vi "Test Summary Page.vi"(8 "error in (no error)":errorcluster, 9 "Test Configuration":T1, 10 "Test Results":T8, 11 "Type":string="Step") -> (0 "error out":errorcluster, 3 "Result":bool)   [LabVIEW 2015]
uses:
  Tests/Controls/Test Results.ctl
  Tests/Controls/Step Result.ctl
  Tests/Controls/Test Configuration.ctl
  Tests/Controls/Vacuum Test.ctl
  Tests/Controls/Test Timing.ctl
  Tests/Controls/Vaccum Thresholds.ctl
  Tests/Controls/Helium Test.ctl
  Tests/Controls/Helium Thresholds.ctl
  Tests/Controls/Functional Test.ctl
panel:
  out "String Result":string
  in  "OK":bool
  in  "Thresholds":i32(listbox)=-1
  # "Test Result Summary"
  # "Result"
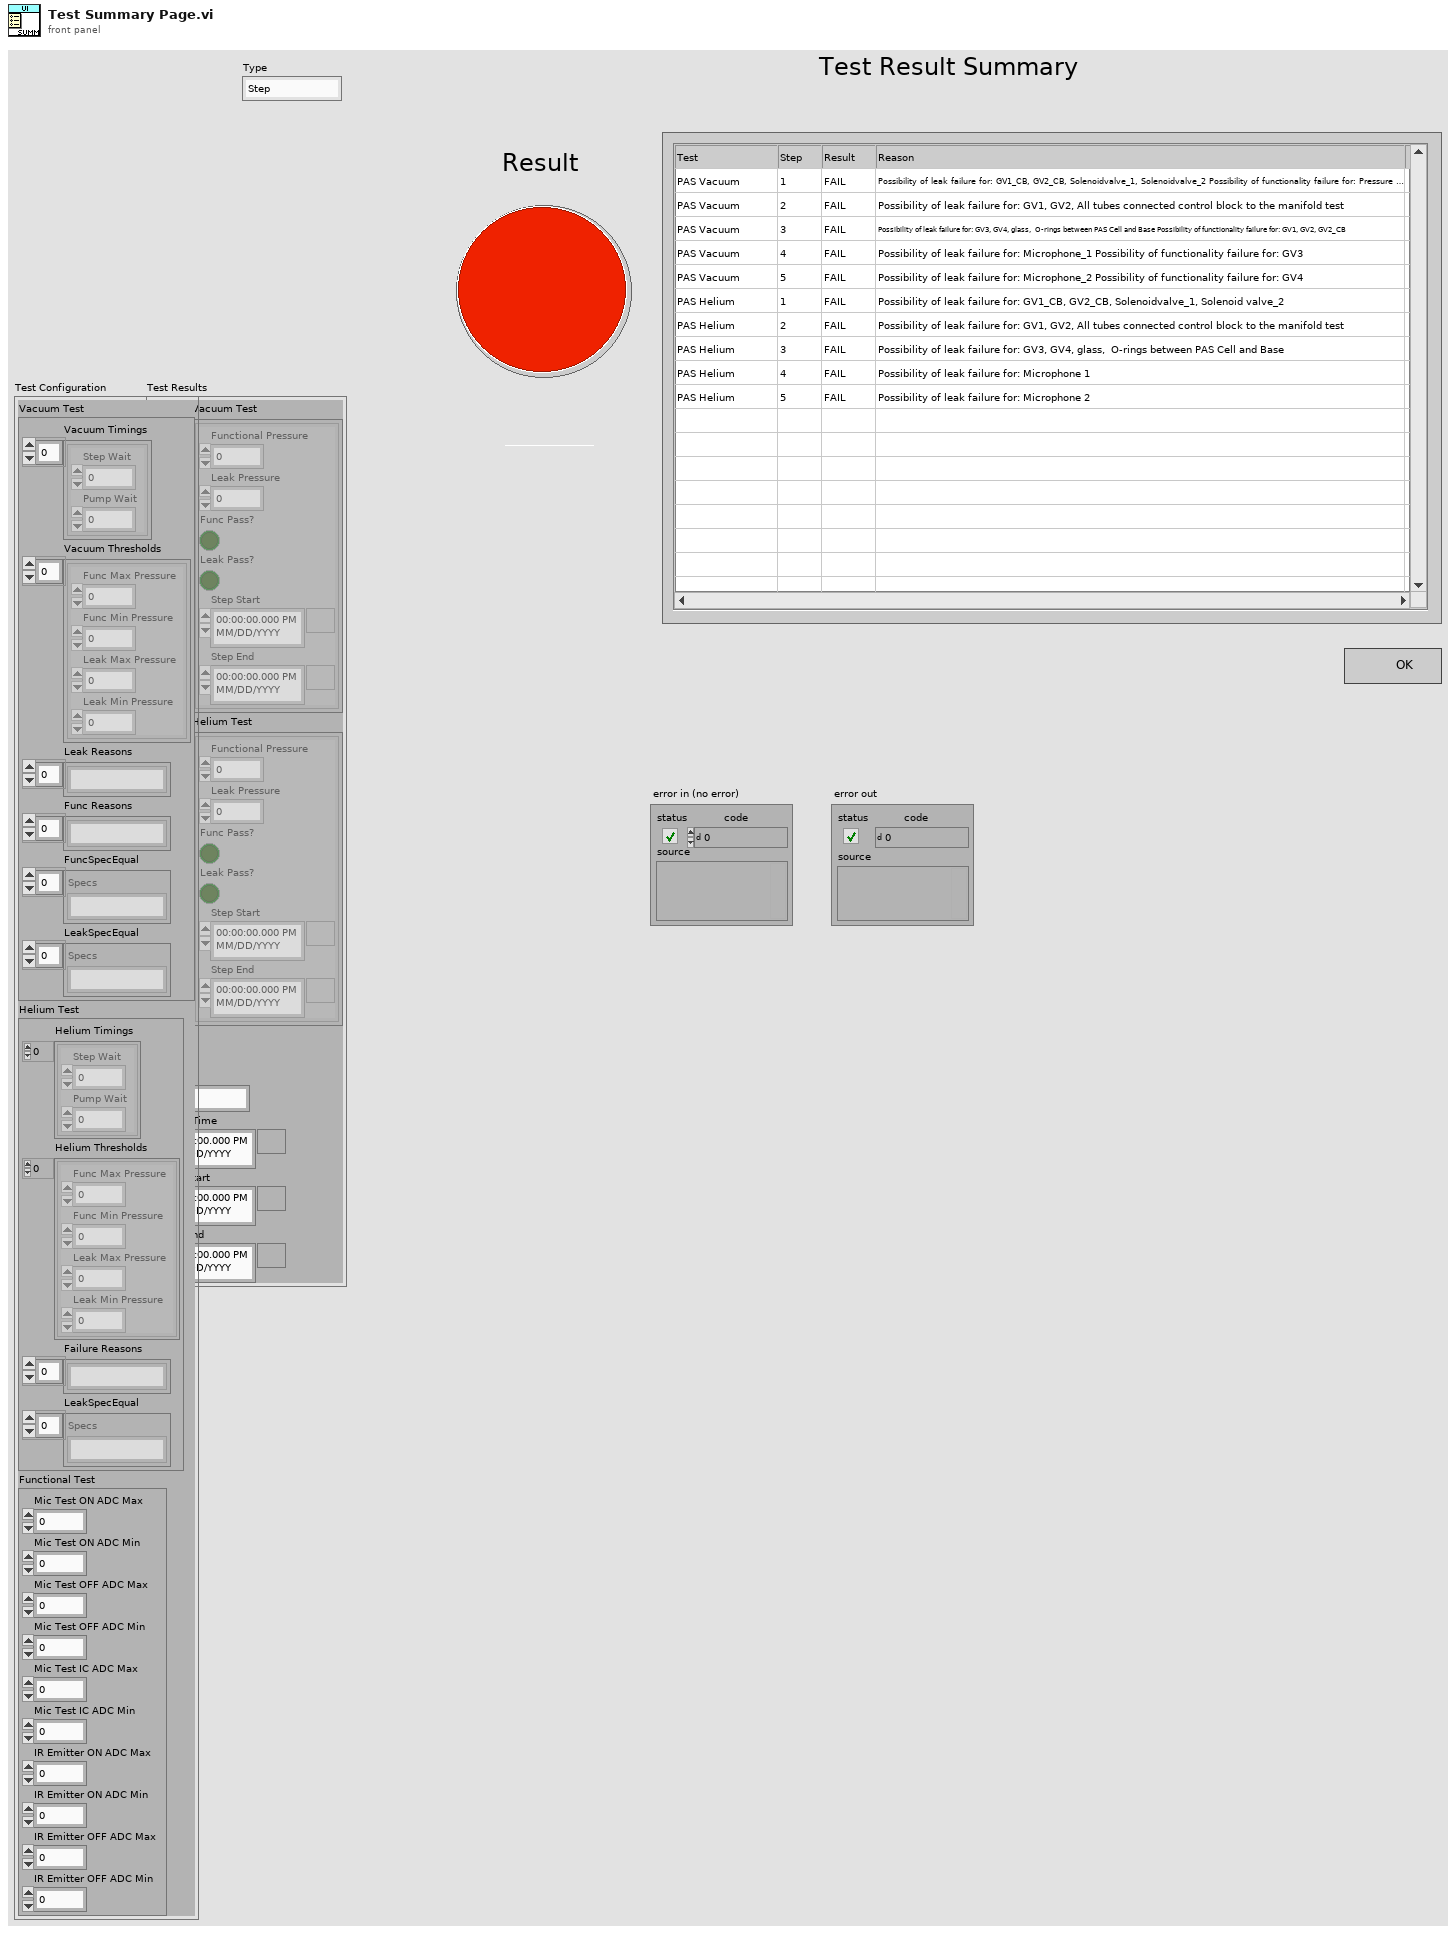
[diagram p1: front panel]
types:
  T1 = typedef "Test Configuration.ctl" = cluster{"Vacuum Test":T2, "Helium Test":T5, "Functional Test":T7}
  T2 = typedef "Vacuum Test.ctl" = cluster{"Vacuum Timings":T3[], "Vacuum Thresholds":T4[], "Leak Reasons":string[], "Func Reasons":string[], "FuncSpecEqual":string[], "LeakSpecEqual":string[]}
  T3 = typedef "Test Timing.ctl" = cluster{"Step Wait":dbl, "Pump Wait":dbl}
  T4 = typedef "Vaccum Thresholds.ctl" = cluster{"Func Max Pressure":dbl, "Func Min Pressure":dbl, "Leak Max Pressure":dbl, "Leak Min Pressure":dbl}
  T5 = typedef "Helium Test.ctl" = cluster{"Helium Timings":T3[], "Helium Thresholds":T6[], "Failure Reasons":string[], "LeakSpecEqual":string[]}
  T6 = typedef "Helium Thresholds.ctl" = cluster{"Func Max Pressure":dbl, "Func Min Pressure":dbl, "Leak Max Pressure":dbl, "Leak Min Pressure":dbl}
  T7 = typedef "Functional Test.ctl" = cluster{"Mic Test ON ADC Max":dbl, "Mic Test ON ADC Min":dbl, "Mic Test OFF ADC Max":dbl, "Mic Test OFF ADC Min":dbl, "Mic Test IC ADC Max":dbl, "Mic Test IC ADC Min":dbl, "IR Emitter ON ADC Max":dbl, "IR Emitter ON ADC Min":dbl, "IR Emitter OFF ADC Max":dbl, "IR Emitter OFF ADC Min":dbl}
  T8 = typedef "Test Results.ctl" = cluster{"Vacuum Test":T9[], "Helium Test":T9[], "Aborted?":bool, "Reason":string, "Abort Time":timestamp, "Test Start":timestamp, "Test End":timestamp}
  T9 = typedef "Step Result.ctl" = cluster{"Functional Pressure":dbl, "Leak Pressure":dbl, "Func Pass?":bool, "Leak Pass?":bool, "Step Start":timestamp, "Step End":timestamp}
  T10 = typedef "LVPoint32TypeDef.ctl" = cluster{"Horizontal":i32, "Vertical":i32}
  T11 = typedef "LVRowAndColumnTypeDef.ctl" = cluster{"Row":i32, "Column":i32}
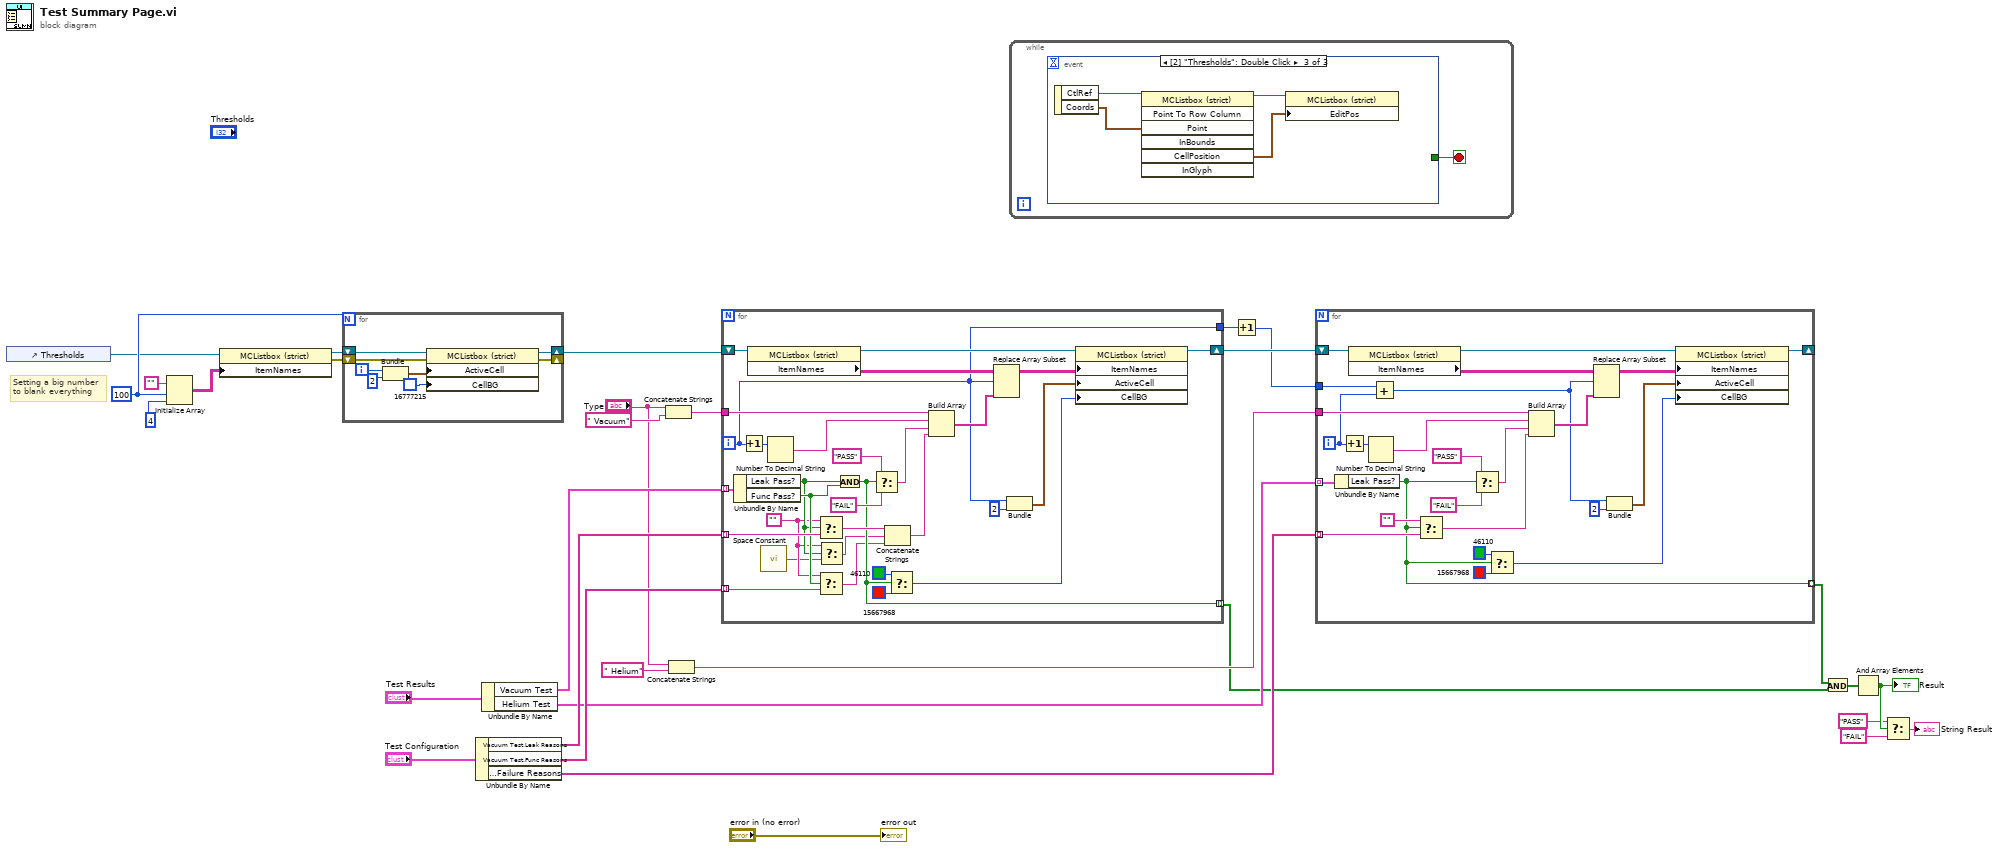
[diagram p0: block diagram]
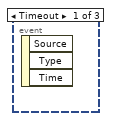
[diagram p2: hidden frame]
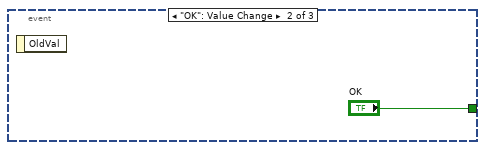
[diagram p3: hidden frame]
diagram:
  w8 = 100 ("dimension size")
  # "Setting a big number\nto blank everything"
  n1 = control-ref of="Thresholds"() -> (w7:refnum<vi>)
  n2 = Initialize Array("", w8, 4 ("dimension size")) -> (w12:string[][])
  n3 = property class="MCListbox (strict)"(reference=w7, "ItemNames"=w12) -> (reference out=w11:refnum<vi>, error out=w10:errorcluster)  [unwired: 1 in]
  n4 = for {
    N: w8 -> [_]
    shift-right: [w38] -> w6
    shift-left: w11 -> [w39]
    shift-right: [w32] -> _
    shift-left: w10 -> [w33]
    i -> [w37]
    n5 = Bundle(w37, "element"=2) -> (w35:cluster{i32, "element":i32})  [unwired: 1 in]
    n6 = property class="MCListbox (strict)"(reference=w39, error in=w33, "ActiveCell"=w35, "CellBG"=u32 16777215) -> (reference out=w38:refnum<vi>, error out=w32:errorcluster)
  }
  n7 = Unbundle By Name("Test Configuration") -> ("Vacuum Test.Leak Reasons"=w27:string[], "Vacuum Test.Func Reasons"=w26:string[], "Helium Test.Failure Reasons"=w21:string[])
  n8 = Unbundle By Name("Test Results") -> ("Vacuum Test"=w31:T9[], "Helium Test"=w22:T9[])
  n9 = Concatenate Strings("Type", " Vacuum") -> (w29:string)
  n10 = Concatenate Strings("Type", " Helium") -> (w23:string)
  n11 = for {
    tunnel: w31 -> [w69] mode=indexing
    tunnel: w29 -> [w65]
    tunnel: w27 -> [w62] mode=indexing
    tunnel: w26 -> [w60] mode=indexing
    shift-right: [w52] -> w25
    shift-left: w6 -> [w57]
    tunnel: [w46] -> w5 mode=indexing
    tunnel: [w45] -> w20
    i -> [w45]
    w42 = ""
    n12 = Unbundle By Name(w69) -> ("Leak Pass?"=w43:bool, "Func Pass?"=w61:bool)
    n13 = Increment(x=w45) -> (x+1=w68:i32)
    n14 = property class="MCListbox (strict)"(reference=w57) -> (reference out=w54:refnum<vi>, "ItemNames"=w56:string[][])  [unwired: 1 in, 1 out]
    n15 = call <vilib>:"Space Constant.vi"() -> ("String"=w41:string)
    n16 = Number To Decimal String(number=w68) -> (decimal integer string=w64:string)  [unwired: 1 in]
    n17 = Select(t=w42, s=w43, f=w62) -> (s? t:f=w59:string)
    n18 = Select(t=w42, s=w61, f=w60) -> (s? t:f=w44:string)
    n19 = Select(t=w42, s=w43, f=w41) -> (s? t:f=w40:string)
    n20 = And(x=w43, y=w61) -> (x .and. y?=w46:bool)
    n21 = Select(t="PASS", s=w46, f="FAIL") -> (s? t:f=w63:string)
    n22 = Concatenate Strings(w59, w40, w44) -> (w58:string)
    n23 = Select(t=u32 46110, s=w46, f=u32 15667968) -> (s? t:f=w47:u32)
    n24 = Build Array(w65, w64, w63, w58) -> (w55:string[])
    n25 = Replace Array Subset(array=w56, new element=w55, index (row)=w45) -> (w53:string[][])  [unwired: 1 in]
    n26 = Bundle(w45, 2) -> (w50:cluster{i32, i32})  [unwired: 1 in]
    n27 = property class="MCListbox (strict)"(reference=w54, "ItemNames"=w53, "ActiveCell"=w50, "CellBG"=w47) -> (reference out=w52:refnum<vi>)  [unwired: 1 in, 1 out]
  }
  n28 = while {
    stop <- w70 stop-if-true
    n29 = event shown="[2] \"Thresholds\": Double Click" {
      selector: _ -> [_ _ _]
      dyn-events: _ -> [_ _ _]
      timeout: _ -> [_ _ _]
      tunnel: [_ "OK" _] -> w70
      event Timeout {
        n30 = event-data() -> ()  [unwired: 1 in, 3 out]
      }
      event "OK": Value Change {
        n31 = event-data() -> ()  [unwired: 1 in, 1 out]
      }
      event "Thresholds": Double Click {
        n32 = event-data() -> ("CtlRef"=w75:refnum<vi>, "Coords"=w74:T10)  [unwired: 1 in]
        n33 = invoke class="MCListbox (strict)" method="Point To Row Column"(reference=w75, "Point"=w74) -> (reference out=w73:refnum<vi>, "CellPosition"=w72:T11)  [unwired: 5 in, 5 out]
        n34 = property class="MCListbox (strict)"(reference=w73, "EditPos"=w72) -> ()  [unwired: 1 in, 2 out]
      }
    }
  }
  n35 = Increment(x=w20) -> (x+1=w19:i32)
  n36 = for {
    tunnel: w22 -> [w100] mode=indexing
    tunnel: w23 -> [w96]
    tunnel: w21 -> [w93] mode=indexing
    shift-right: [w87] -> _
    shift-left: w25 -> [w92]
    tunnel: [w80] -> w18 mode=indexing
    tunnel: w19 -> [w78]
    i -> [w77]
    n37 = Unbundle By Name(w100) -> ("Leak Pass?"=w80:bool)
    n38 = Increment(x=w77) -> (x+1=w99:i32)
    n39 = property class="MCListbox (strict)"(reference=w92) -> (reference out=w89:refnum<vi>, "ItemNames"=w91:string[][])  [unwired: 1 in, 1 out]
    n40 = Number To Decimal String(number=w99) -> (decimal integer string=w95:string)  [unwired: 1 in]
    n41 = Add(x=w78, y=w77) -> (x+y=w76:i32)
    n42 = Select(t="", s=w80, f=w93) -> (s? t:f=w79:string)
    n43 = Select(t="PASS", s=w80, f="FAIL") -> (s? t:f=w94:string)
    n44 = Select(t=u32 46110, s=w80, f=u32 15667968) -> (s? t:f=w82:u32)
    n45 = Build Array(w96, w95, w94, w79) -> (w90:string[])
    n46 = Replace Array Subset(array=w91, new element=w90, index (row)=w76) -> (w88:string[][])  [unwired: 1 in]
    n47 = Bundle(w76, 2) -> (w85:cluster{i32, i32})  [unwired: 1 in]
    n48 = property class="MCListbox (strict)"(reference=w89, "ItemNames"=w88, "ActiveCell"=w85, "CellBG"=w82) -> (reference out=w87:refnum<vi>)  [unwired: 1 in, 1 out]
  }
  n49 = And(x=w18, y=w5) -> (x .and. y?=w17:bool[])
  n50 = And Array Elements(Boolean array=w17) -> (logical AND=w4:bool)
  "Result" <- w4
  n51 = Select(t="PASS", s=w4, f="FAIL") -> (s? t:f=→"String Result":string)
  "error out" <- "error in (no error)"
